vi "HK Channel Read Channels.vi"(8 "error in (no error)":errorcluster, 11 "HK Channel in":refnum<class "HK Table.lvclass">) -> (0 "error out":errorcluster, 3 "HK Channel out":refnum<class "HK Table.lvclass">)   [LabVIEW 2024, in "HK Table.lvclass"]
uses:
  HK Table.lvclass
  HK Table.lvclass/HK Table.ctl
  HK Item/HK Item.lvclass
  HK Alarms/HK Alarms.lvclass
  HK Item/HK Item.lvclass/HK Item.ctl
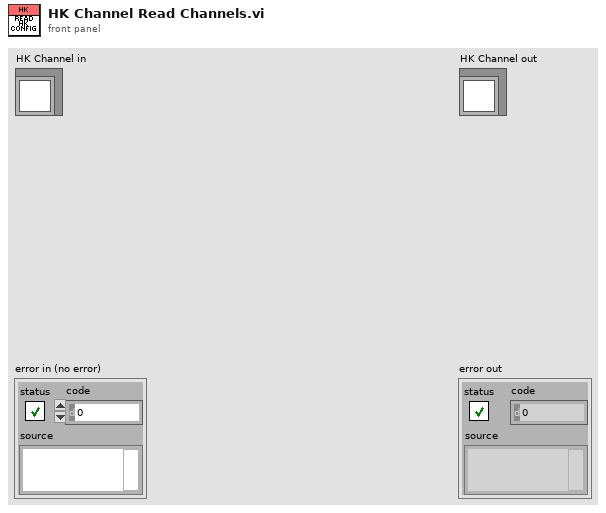
[diagram p1: front panel]
types:
  T1 = typedef "HK Table.lvclass/HK Channel Settings.ctl" = cluster{"Name":string, "Channel Setup":T2, "Value":dbl, "Timestamp":timestamp, "Scaling":T4, "Physical":T6, "Limits":T7, "Alarms":T8[]}
  T2 = typedef "HK Item.lvclass/HK Channel Units and Setup.ctl" = cluster{"Unit Type":string, "Units":string, "Configuration":string, "Digits":i32, "Data Type":T3, "Exponential?":bool, "Source":string}
  T3 = typedef "HK Item.lvclass/HK Channel enum Data Type.ctl" = enum16{"Floating Point", "Integer", "Enum", "String", "Waveform", "File"}
  T4 = typedef "HK Item.lvclass/HK Channel Settings Scaling.ctl" = cluster{"Scaling Type":T5, "Parameters":dbl[]}
  T5 = typedef "HK Item.lvclass/HK Channel enum Scaling Type.ctl" = enum16{"None", "Polynomial"}
  T6 = typedef "HK Item.lvclass/HK Channel Settings Physical.ctl" = cluster{"Type":string, "Device":string, "Module":string, "Channel":i32}
  T7 = typedef "HK Item.lvclass/HK Channel Settings Limits.ctl" = cluster{"Low Red":dbl, "Low Yellow":dbl, "Hi Yellow":dbl, "Hi Red":dbl}
  T8 = typedef "HK Item.lvclass/HK Channel Settings Alarms.ctl" = cluster{"Enabled":bool, "Deadband":i32, "Action":T9}
  T9 = typedef "HK Item.lvclass/HK Alarm enum Action.ctl" = enum16{"Light", "Message", "Safe"}
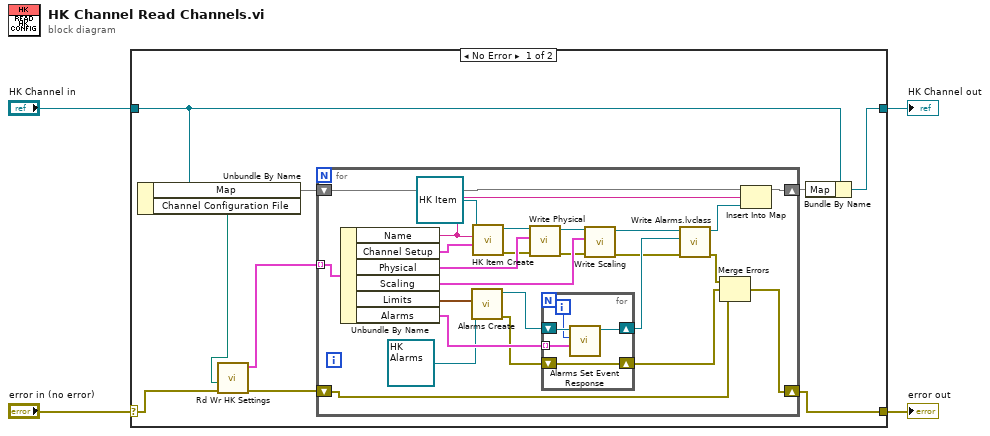
[diagram p0: block diagram]
diagram:
  n1 = case shown="No Error" "error in (no error)" {
    selector: "error in (no error)" -> [w13 w45]
    tunnel: [w7 w45] -> w3
    tunnel: [w12 w44] -> w1
    tunnel: "HK Channel in" -> [w10 w44]
    frame No Error {
      n2 = Unbundle By Name(w10) -> ("Map"=w9:map{string, refnum<class "HK Item.lvclass">}, "Channel Configuration File"=w5:path)
      n3 = call "Rd Wr HK Settings.vi"("error in (no error)"=w13, "File Path"=w5) -> ("error out"=w8:errorcluster, "channels"=w11:T1[])  [unwired: 8 in]
      n4 = for {
        tunnel: w11 -> [w37] mode=indexing
        shift-right: [w36] -> w6
        shift-left: w9 -> [w38]
        shift-right: [w16] -> w7
        shift-left: w8 -> [w17]
        n5 = Unbundle By Name(w37) -> ("Name"=w35:string, "Channel Setup"=w34:T2, "Physical"=w32:T6, "Scaling"=w30:T4, "Limits"=w29:T7, "Alarms"=w27:T8[])
        n6 = call-dynamic "Alarms Create.vi"("Limits"=w29, "Alarms in"=refnum<class "HK Alarms.lvclass"> refnum) -> ("error out"=w20:errorcluster, "Alarms out"=w28:refnum<class "HK Alarms.lvclass">)  [unwired: 8 in]
        n7 = call-dynamic "HK Item Create.vi"("Channel Setup"=w34, "Name"=w35, "HK Item in"=refnum<class "HK Item.lvclass"> refnum) -> ("error out"=w23:errorcluster, "HK Item out"=w33:refnum<class "HK Item.lvclass">)  [unwired: 7 in]
        n8 = call "Write Physical.vi"("error in (no error)"=w23, "Physical"=w32, "HK Item in"=w33) -> ("error out"=w22:errorcluster, "HK Item out"=w31:refnum<class "HK Item.lvclass">)  [unwired: 7 in]
        n9 = for {
          shift-right: [w40] -> w25
          shift-left: w28 -> [w43]
          tunnel: w27 -> [w41] mode=indexing
          shift-right: [w39] -> w18
          shift-left: w20 -> [w39]
          i -> [w42]
          n10 = call-dynamic "Alarms Set Event Response.vi"("Alarms"=w41, "Alarm Event"=w42, "Alarms in"=w43) -> ("Alarms out"=w40:refnum<class "HK Alarms.lvclass">)  [unwired: 7 in, 1 out]
        }
        n11 = call "Write Scaling.vi"("error in (no error)"=w22, "Scaling"=w30, "HK Item in"=w31) -> ("error out"=w21:errorcluster, "HK Item out"=w26:refnum<class "HK Item.lvclass">)  [unwired: 7 in]
        n12 = call "Write Alarms.lvclass.vi"("error in (no error)"=w21, "Alarms.lvclass"=w25, "HK Item in"=w26) -> ("error out"=w19:errorcluster, "HK Item out"=w24:refnum<class "HK Item.lvclass">)  [unwired: 7 in]
        n13 = Merge Errors(w19, w18, w17) -> (w16:errorcluster)
        n14 = Insert Into Map(map in=w38, key=w35, value=w24) -> (map out=w36:map{string, refnum<class "HK Item.lvclass">})  [unwired: 2 out]
      }
      n15 = Bundle By Name(cluster=w10, "Map"=w6) -> (w12:refnum<class "HK Table.lvclass">)
    }
    frame Error {
    }
  }
  "error out" <- w3
  "HK Channel out" <- w1
